vi "scoop_driver_main.vi"() -> ()   [LabVIEW 2026]
panel:
  out "String":string
  in  "VISA resource name":refnum<visa-resource-name>
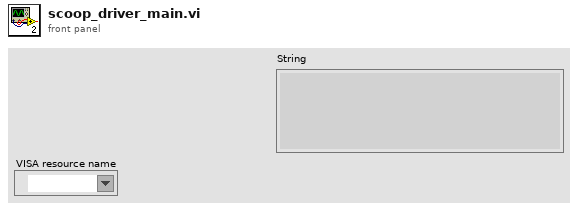
[diagram p1: front panel]
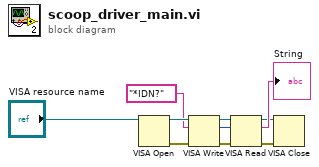
[diagram p0: block diagram]
diagram:
  n1 = VISA Open(VISA resource name="VISA resource name") -> (VISA resource name=w9:refnum<visa-resource-name>, error out=w8:errorcluster)  [unwired: 4 in]
  n2 = VISA Write(VISA resource name=w9, write buffer="*IDN?", error in (no error)=w8) -> (VISA resource name out=w3:refnum<visa-resource-name>, return count=w2:u32, error out=w1:errorcluster)
  n3 = VISA Read(VISA resource name=w3, byte count=w2, error in (no error)=w1) -> (VISA resource name out=w5:refnum<visa-resource-name>, read buffer=→"String":string, error out=w4:errorcluster)  [unwired: 1 out]
  n4 = VISA Close(VISA resource name=w5, error in (no error)=w4) -> ()  [unwired: 1 out]
